vi "GNSS1-SET-2.vi"(0 "开机时间":refnum<vi>, 1 "bd卫星数":refnum<vi>, 2 "spare":refnum<vi>, 3 "glo时间差":refnum<vi>, 4 "glo卫星数":refnum<vi>, 5 "glo北京时间":refnum<vi>, 6 "glo故障字":refnum<vi>, 7 "glo速度位置":refnum<vi>, 10 "glo定位状态":refnum<vi>, 11 "glo收星数":refnum<vi>, 12 "软件版本":refnum<vi>, 13 "glo-pdop":refnum<vi>) -> (14 "添加的数组2":u8[](array[numeric]))   [LabVIEW 2012]
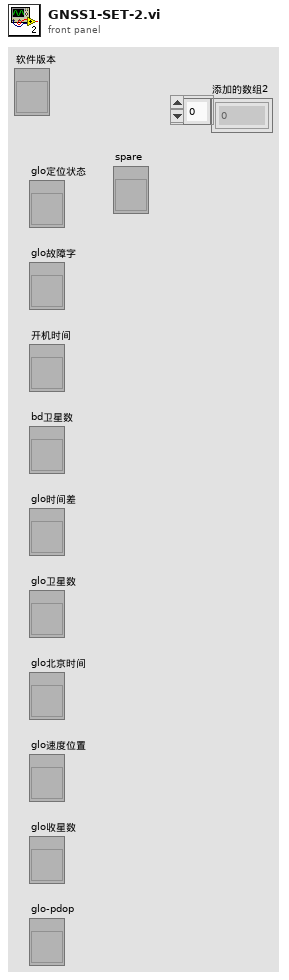
[diagram p1: front panel]
types:
  T1 = cluster{"GLO北向速度":sgl, "GLO东向速度":sgl, "GLO天向速度":sgl, "GLO经度":sgl, "GLO纬度":sgl, "GLO高度":sgl}
  T2 = typedef "LVDateTimeRec.ctl" = cluster{"秒数的小数部分":dbl, "秒":i32, "分":i32, "时":i32, "日":i32, "月":i32, "年":i32, "天数（周）":i32, "天数（年）":i32, "DST":i32}
  T3 = enum8{"无故障", "未正常初始化时间", "PDOP值>12", "没有可用卫星", "只有1颗可用卫星", "只有2颗可用卫星", "只有3颗可用卫星", "观测矩阵不可求逆", "定位解算不收敛", "高程超差", "速度大于10km/s"}
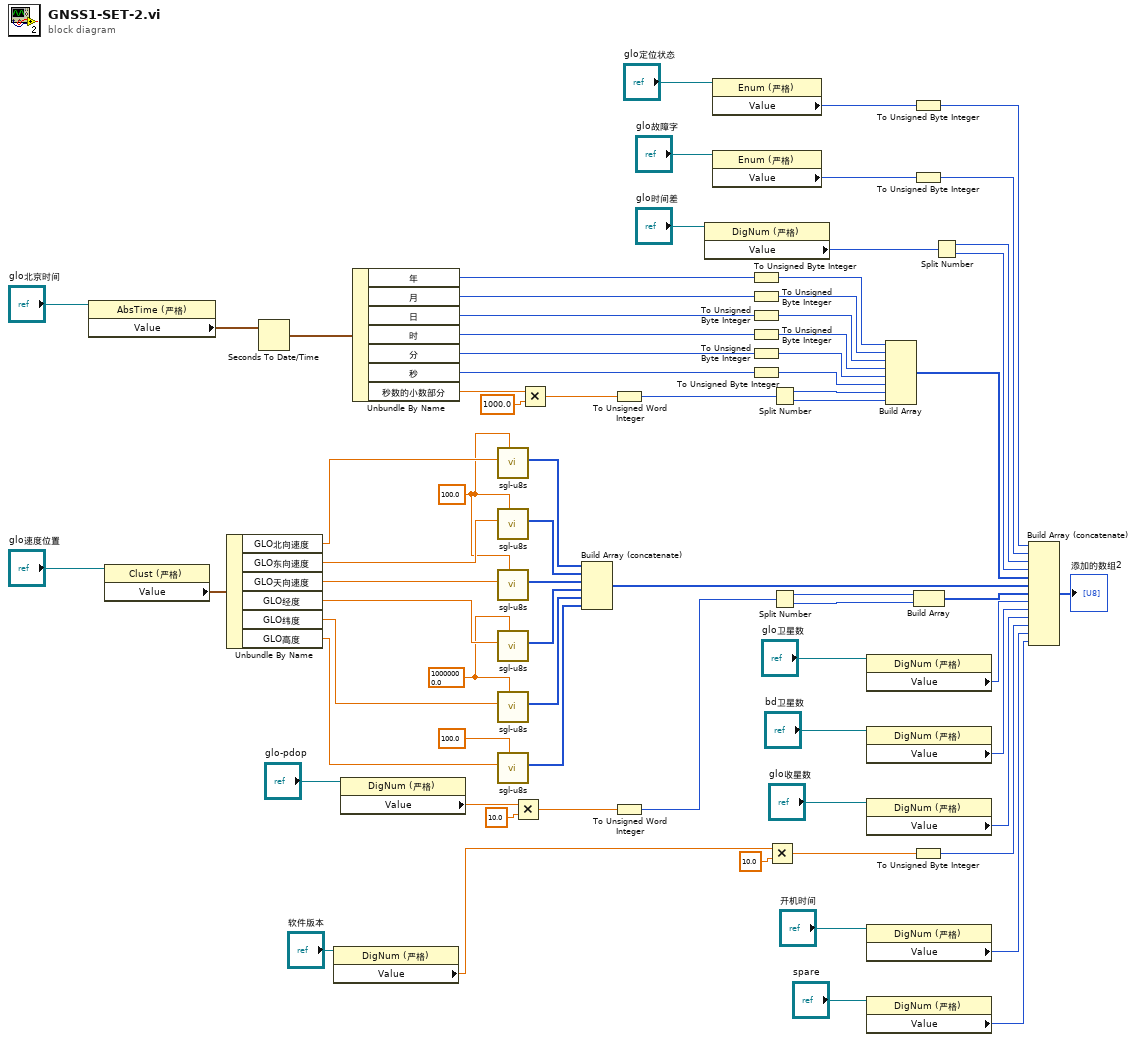
[diagram p0: block diagram]
diagram:
  w28 = sgl 10000000.0 ("精度")
  w29 = sgl 100.0 ("y")
  n1 = property on="属性节点" class="AbsTime (严格)"(reference="glo北京时间") -> ("Value"=w63:timestamp)  [unwired: 1 in, 2 out]
  n2 = property on="属性节点" class="Clust (严格)"(reference="glo速度位置") -> ("Value"=w64:T1)  [unwired: 1 in, 2 out]
  n3 = Unbundle By Name(w64) -> ("GLO北向速度"=w36:sgl, "GLO东向速度"=w34:sgl, "GLO天向速度"=w33:sgl, "GLO经度"=w32:sgl, "GLO纬度"=w31:sgl, "GLO高度"=w30:sgl)
  n4 = Seconds To Date/Time(time stamp (now)=w63) -> (date time rec=w56:T2)  [unwired: 1 in]
  n5 = property class="DigNum (严格)"(reference="软件版本") -> ("Value"=w2:sgl)  [unwired: 1 in, 2 out]
  n6 = property on="属性节点" class="DigNum (严格)"(reference="glo-pdop") -> ("Value"=w65:sgl)  [unwired: 1 in, 2 out]
  n7 = Unbundle By Name(w56) -> ("年"=w55:i32, "月"=w53:i32, "日"=w52:i32, "时"=w51:i32, "分"=w50:i32, "秒"=w49:i32, "秒数的小数部分"=w48:dbl)
  n8 = call "sgl-u8s.vi"("输入sgl"=w36, "精度"=w29) -> ("u8s"=w35:u8[])  [unwired: 8 in]
  n9 = call "sgl-u8s.vi"("输入sgl"=w34, "精度"=w29) -> ("u8s"=w27:u8[])  [unwired: 8 in]
  n10 = call "sgl-u8s.vi"("输入sgl"=w33, "精度"=w29) -> ("u8s"=w26:u8[])  [unwired: 8 in]
  n11 = call "sgl-u8s.vi"("输入sgl"=w32, "精度"=w28) -> ("u8s"=w25:u8[])  [unwired: 8 in]
  n12 = call "sgl-u8s.vi"("输入sgl"=w31, "精度"=w28) -> ("u8s"=w24:u8[])  [unwired: 8 in]
  n13 = call "sgl-u8s.vi"("输入sgl"=w30, "精度"=sgl 100.0) -> ("u8s"=w23:u8[])  [unwired: 8 in]
  n14 = Multiply(x=w65, y=sgl 10.0) -> (x*y=w20:sgl)
  n15 = Multiply(x=w48, y=1000.0) -> (x*y=w46:dbl)
  n16 = Build Array (concatenate)(w35, w27, w26, w25, w24, w23) -> (w22:u8[])
  n17 = To Unsigned Word Integer(number=w46) -> (unsigned 16bit integer=w45:u16)
  n18 = To Unsigned Word Integer(number=w20) -> (unsigned 16bit integer=w17:u16)
  n19 = property on="属性节点" class="DigNum (严格)"(reference="glo时间差") -> ("Value"=w62:u16)  [unwired: 1 in, 2 out]
  n20 = property on="属性节点" class="Enum (严格)"(reference="glo定位状态") -> ("Value"=w59:enum8{"无效", "GLO定位", "GLO+BD定位", "BD定位"})  [unwired: 1 in, 2 out]
  n21 = property on="属性节点" class="Enum (严格)"(reference="glo故障字") -> ("Value"=w60:T3)  [unwired: 1 in, 2 out]
  n22 = To Unsigned Byte Integer(number=w55) -> (unsigned 8bit integer=w54:u8)
  n23 = To Unsigned Byte Integer(number=w53) -> (unsigned 8bit integer=w44:u8)
  n24 = To Unsigned Byte Integer(number=w52) -> (unsigned 8bit integer=w43:u8)
  n25 = To Unsigned Byte Integer(number=w51) -> (unsigned 8bit integer=w42:u8)
  n26 = To Unsigned Byte Integer(number=w50) -> (unsigned 8bit integer=w41:u8)
  n27 = To Unsigned Byte Integer(number=w49) -> (unsigned 8bit integer=w40:u8)
  n28 = Multiply(x=w2, y=sgl 10.0) -> (x*y=w69:sgl)
  n29 = Split Number(x=w45) -> (hi(x)=w39:u8, lo(x)=w38:u8)
  n30 = Split Number(x=w17) -> (hi(x)=w19:u8, lo(x)=w18:u8)
  n31 = property on="属性节点" class="DigNum (严格)"(reference="glo卫星数") -> ("Value"=w66:u8)  [unwired: 1 in, 2 out]
  n32 = property on="属性节点" class="DigNum (严格)"(reference="bd卫星数") -> ("Value"=w67:u8)  [unwired: 1 in, 2 out]
  n33 = property on="属性节点" class="DigNum (严格)"(reference="glo收星数") -> ("Value"=w68:u8)  [unwired: 1 in, 2 out]
  n34 = property on="属性节点" class="DigNum (严格)"(reference="开机时间") -> ("Value"=w72:u8)  [unwired: 1 in, 2 out]
  n35 = property on="属性节点" class="DigNum (严格)"(reference="spare") -> ("Value"=w4:u8)  [unwired: 1 in, 2 out]
  n36 = Build Array(w54, w44, w43, w42, w41, w40, w39, w38) -> (w37:u8[])
  n37 = To Unsigned Byte Integer(number=w59) -> (unsigned 8bit integer=w15:u8)
  n38 = To Unsigned Byte Integer(number=w60) -> (unsigned 8bit integer=w61:u8)
  n39 = To Unsigned Byte Integer(number=w69) -> (unsigned 8bit integer=w71:u8)
  n40 = Build Array(w19, w18) -> (w16:u8[])
  n41 = Split Number(x=w62) -> (hi(x)=w58:u8, lo(x)=w57:u8)
  n42 = Build Array (concatenate)(w15, w61, w58, w57, w37, w22, w16, w66, w67, w68, w71, w72, w4) -> (→"添加的数组2":u8[])
